vi "Read Discrete from Slave.vi"(7 "Unit ID":u8, 8 "error in (no error)":errorcluster, 9 "length":u16, 10 "start":u16, 11 "Modbus Master in":refnum<class "Modbus Master.lvclass">) -> (0 "error out":errorcluster, 3 "discrete inputs":bool[](array[boolean]))   [LabVIEW 2020, in "Modbus Master Engine.lvlib"]
uses:
  Modbus Master Engine.lvlib
  API/Master/Modbus Master.lvclass
  C:/Users/Administrator/Desktop/GIT/Modbus-Custom-Device-v2/Source/Custom Device Support/API/Modbus API.lvclass
  API/Modbus API.lvclass/Modbus API.ctl
  Transmission Data Unit/Transmission Data Unit.lvclass/Transmission Data Unit.ctl
  Transmission Data Unit/Write Unit ID.vi
  API/Read Transmission Data Unit.vi
  API/Write Transmission Data Unit.vi
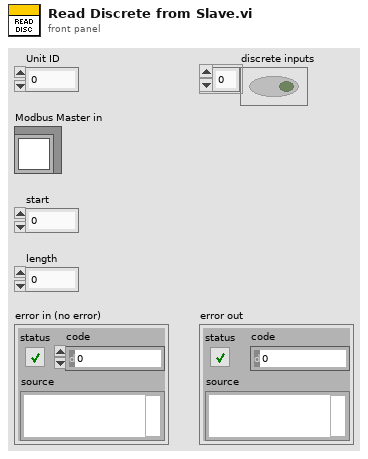
[diagram p1: front panel]
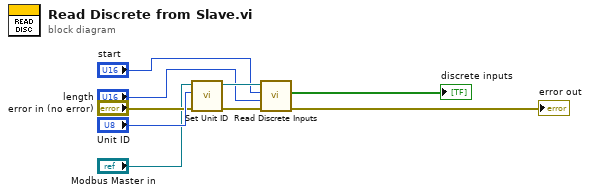
[diagram p0: block diagram]
diagram:
  n1 = call "Set Unit ID.vi"("error in"="error in (no error)", "unit ID"="Unit ID", "Modbus master in"="Modbus Master in") -> ("error out"=w8:errorcluster, "Modbus master out"=w6:refnum<class "Modbus Master.lvclass">)  [unwired: 7 in]
  n2 = call-dynamic "Read Discrete Inputs.vi"("error in"=w8, "number of inputs"="length", "starting address"="start", "Modbus master in"=w6) -> ("error out"=→"error out":errorcluster, "discrete inputs"=→"discrete inputs":bool[])  [unwired: 5 in, 1 out]
